vi "실습 2-2.vi"() -> ()   [LabVIEW 2014]
panel:
  out "큐 데이터 출력":string
  in  "정지":bool
  in  "Enqueue":bool
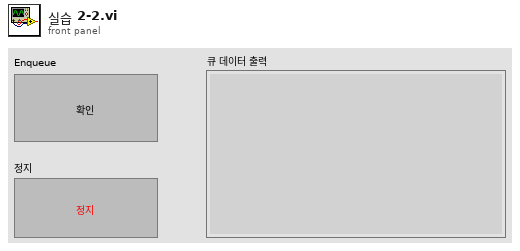
[diagram p1: front panel]
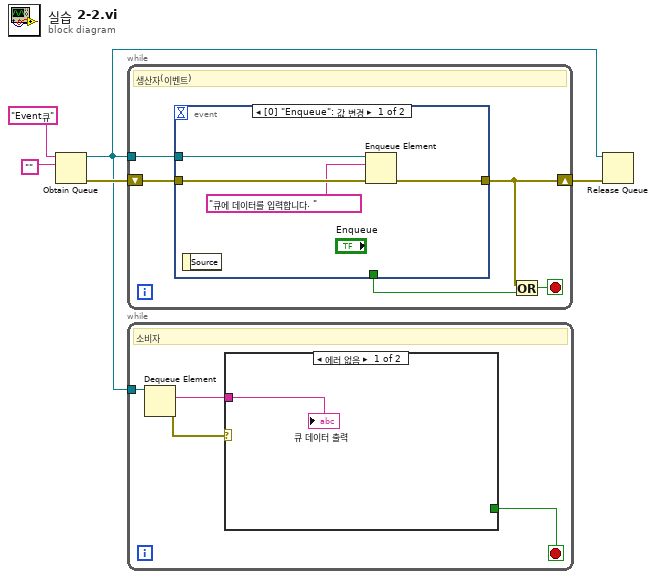
[diagram p0: block diagram]
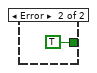
[diagram p2: hidden frame]
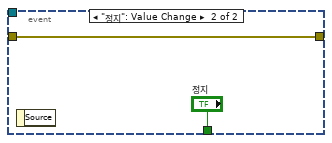
[diagram p3: hidden frame]
diagram:
  n1 = Obtain Queue(name (unnamed)="Event큐" ("이름(이름없음)"), element data type="") -> (queue out=w1:refnum<queue>, error out=w5:errorcluster)  [unwired: 3 in, 1 out]
  n2 = while {
    shift-right: [w7] -> w4
    shift-left: w5 -> [w10]
    tunnel: w1 -> [w6]
    stop <- w8 stop-if-true
    # "생산자(이벤트)"
    n3 = event shown="[0] \"Enqueue\": 값 변경" {
      selector: _ -> [_ _]
      dyn-events: _ -> [_ _]
      timeout: _ -> [_ _]
      tunnel: w10 -> [w14 w16]
      tunnel: [w13 w16] -> w7
      tunnel: [_ "정지"] -> w9
      tunnel: w6 -> [w11 _]
      event "Enqueue": Value Change {
        n4 = event-data() -> ()  [unwired: 1 in, 1 out]
        n5 = Enqueue Element(queue=w11, element="큐에 데이터를 입력합니다. " ("원소"), error in (no error)=w14) -> (error out=w13:errorcluster)  [unwired: 1 in, 2 out]
      }
      event "정지": Value Change {
        n6 = event-data() -> ()  [unwired: 1 in, 1 out]
      }
    }
    n7 = Or(x=w7, y=w9) -> (x .or. y?=w8:bool)
  }
  n8 = while {
    tunnel: w1 -> [w20]
    stop <- w17 stop-if-true
    # "소비자"
    n9 = Dequeue Element(queue=w20) -> (element=w18:string, error out=w19:errorcluster)  [unwired: 2 in, 2 out]
    n10 = case shown="에러 없음" w19 {
      tunnel: w18 -> [w21 _]
      tunnel: [_ TRUE] -> w17
      frame No Error {
        "큐 데이터 출력" <- w21
      }
      frame Error {
      }
    }
  }
  n11 = Release Queue(queue=w1, error in (no error)=w4) -> ()  [unwired: 1 in, 3 out]
